vi "Bowl Feeder Loop.vi"(8 "error in (no error)":errorcluster) -> (0 "error out":errorcluster)   [LabVIEW 2021]
uses:
  Global Variables/FPGA GV.vi
  Global Variables/RT GV.vi
  <vilib>/Utility/error.llb/Error Cluster From Error Code.vi
  <vilib>/rvi/errors/niLvFpgaAdjustHostInterfaceError.vi
  <vilib>/rvi/interface/nirviReadWriteControl/nirviReadWriteControl.xnode
  <vilib>/rvi/interface/Simulation/niFpgaSimulationCallBeginRW.vi
  NiFpgaLv.dll
panel:
  in  "Stop Button":bool
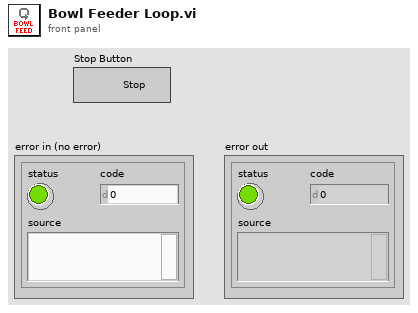
[diagram p1: front panel]
types:
  T1 = cluster{"TL_Red":bool, "TL_Orange":bool, "TL_Green":bool, "TL_Buzzer":bool, "Vaccuum ON":bool, "Vaccuum OFF":bool, "Beckhoff Data":bool, "SOL_Singling":bool, "Bowl Feeder_ ON1":bool, "Buffer 1":bool, "SOL_Pick_Place_Vertical":bool, "SOL_Tube_Feed_Agitatator":bool, "SOL_Tube_Feed_Gating_CYL":bool, "SOL_Insertion _CYL":bool, "SOL_Insertion_Clamp_CYL":bool, "SOL_Cutting_CYL":bool, "SOL_Cutting_Clamp_CYL":bool, "SOL_Insertion_Air_Nozzle":bool, "SOL_Measurement_CYL":bool, "SOL_Pick_Place_Rotary":bool, "SOL_Rejection CYL_1":bool, "SOL_Rejection CYL_2":bool, "SOL_Rejection CYL_3":bool, "SOL_Rejection CYL_4":bool, "Bowl Feeder_ON2":bool, "Linear Feeder 1":bool, "Linear Feeder 2":bool, "Buffer 2":bool, "Buffer 3":bool, "Buffer 4":bool, "Buffer 5":bool, "Buffer 6":bool}
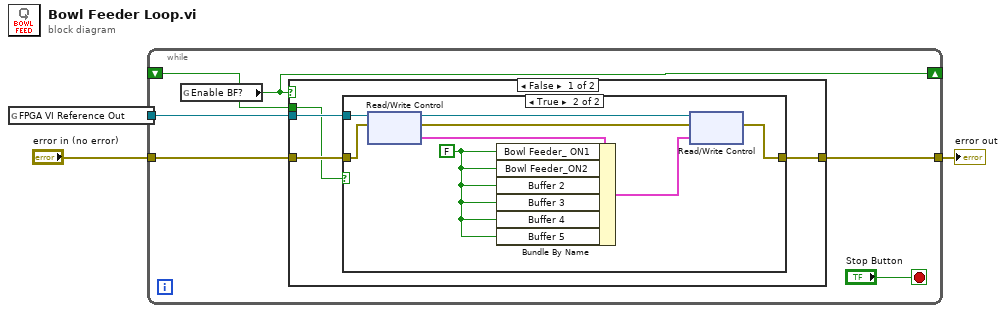
[diagram p0: block diagram]
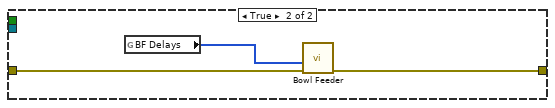
[diagram p3: hidden frame]
diagram:
  n1 = global read "FPGA GV.vi" "FPGA VI Reference Out"() -> (w1:refnum<k20>)
  n2 = while {
    tunnel: "error in (no error)" -> [w9]
    tunnel: [w8] -> w2
    shift-right: [w7] -> _
    shift-left: _ -> [w6]
    tunnel: w1 -> [w5]
    stop <- "Stop Button" stop-if-true
    n3 = global read "RT GV.vi" "Enable BF?"() -> (w7:bool)
    n4 = case shown="False" w7 {
      tunnel: w9 -> [w13 w25]
      tunnel: [w12 w24] -> w8
      tunnel: w6 -> [w10 _]
      tunnel: w5 -> [w11 _]
      frame False {
        n5 = case shown="True" w10 {
          tunnel: w13 -> [w14 w17]
          tunnel: [w14 w16] -> w12
          tunnel: w11 -> [_ w15]
          frame False {
          }
          frame True {
            w18 = FALSE ("SOL_Index_Rotary_CW")
            n6 = xnode "Read/Write Control"("FPGA VI Reference In"=w15, "error in"=w17) -> ("FPGA VI Reference Out"=w19:refnum<k20>, "error out"=w20:errorcluster, "DO 1"=w21:T1)
            n7 = Bundle By Name(cluster=w21, "Bowl Feeder_ ON1"=w18, "Bowl Feeder_ON2"=w18, "Buffer 2"=w18, "Buffer 3"=w18, "Buffer 4"=w18, "Buffer 5"=w18) -> (w22:T1)
            n8 = xnode "Read/Write Control"("FPGA VI Reference In"=w19, "error in"=w20, "DO 1"=w22) -> ("error out"=w16:errorcluster)  [unwired: 1 out]
          }
        }
      }
      frame True {
        n9 = global read "RT GV.vi" "BF Delays"() -> (w23:u32[])
        n10 = call "Bowl Feeder.vi"("error in (no error)"=w25, "BF Delays"=w23) -> ("error out"=w24:errorcluster)  [unwired: 8 in, 1 out]
      }
    }
  }
  "error out" <- w2
